vi "Set Socket.vi"(8 "error in (no error)":errorcluster, 11 "Channel Req in":refnum<class "Channel Req.lvclass">) -> (0 "error out":errorcluster, 3 "Channel Req out":refnum<class "Channel Req.lvclass">)   [LabVIEW 2018, in "Channel Req.lvclass"]
uses:
  Channel Req.lvclass
  Socket2/Socket2/Socket2.lvclass
  Communication Channel/Communication Channel Folder/Communication Channel.lvclass
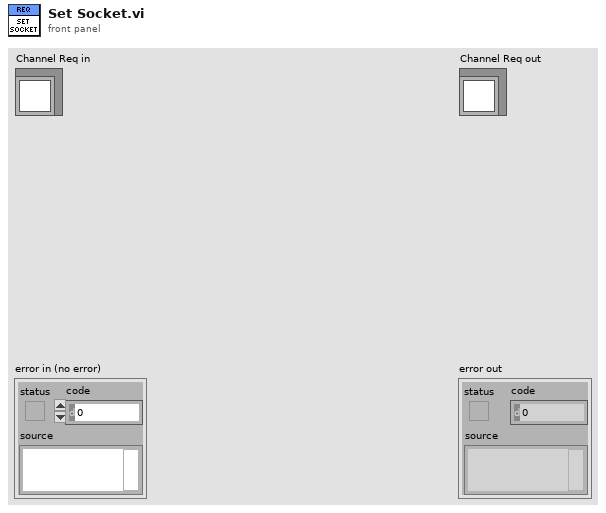
[diagram p1: front panel]
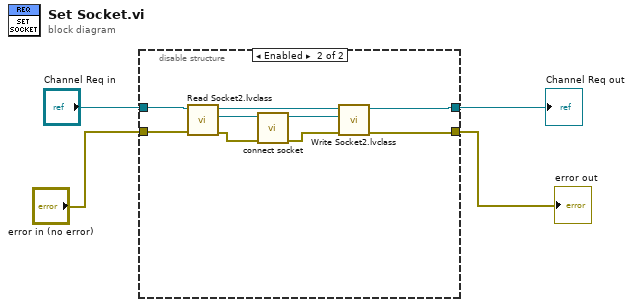
[diagram p0: block diagram]
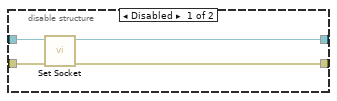
[diagram p2: hidden frame]
diagram:
  n1 = disable-structure shown="Enabled" {
    disable-tunnel: [w8 w9] -> w4
    disable-tunnel: [w7 w10] -> w3
    disable-tunnel: "error in (no error)" -> [w6 w11]
    disable-tunnel: "Channel Req in" -> [w5 w12]
    frame Disabled {
      n2 = call-parent "Set Socket.vi"("error in (no error)"=w6, "Communication Channel in"=w5) -> ("error out"=w8:errorcluster, "Communication Channel out"=w7:refnum<class "Channel Req.lvclass">)  [unwired: 8 in]
    }
    frame Enabled {
      n3 = call-dynamic "Read Socket2.lvclass.vi"("error in (no error)"=w11, "Communication Channel in"=w12) -> ("error out"=w17:errorcluster, "Socket2.lvclass"=w16:refnum<class "Socket2.lvclass">, "Communication Channel out"=w15:refnum<class "Channel Req.lvclass">)  [unwired: 7 in]
      n4 = call "connect socket.vi"("error in (no error)"=w17, "Socket in"=w16) -> ("error out"=w13:errorcluster, "Socket out"=w14:refnum<class "Socket2.lvclass">)  [unwired: 8 in]
      n5 = call-dynamic "Write Socket2.lvclass.vi"("error in (no error)"=w13, "Socket2.lvclass"=w14, "Communication Channel in"=w15) -> ("error out"=w9:errorcluster, "Communication Channel out"=w10:refnum<class "Channel Req.lvclass">)  [unwired: 7 in]
    }
  }
  "error out" <- w4
  "Channel Req out" <- w3
